vi "DSF.Engine.Transceiver.Initialize.vi"(8 "error in (no error)":errorcluster, 9 "transceiver settings":T1, 10 "Transfer Groups Configurations":refnum<class "DSF.Shared.Configuration.Transfer Group.lvclass">[](array[class]), 11 "Transceiver in":refnum<class "DSF.Transceiver.PXImc.lvclass">) -> (0 "error out":errorcluster, 3 "Transceiver out":refnum<class "DSF.Transceiver.PXImc.lvclass">)   [LabVIEW 2018, in "DSF.Transceiver.PXImc.lvlib" / "DSF.Transceiver.PXImc.lvclass"]
uses:
  DSF.Transceiver.PXImc.lvclass
  dsf core/Built/Engine/DSF.Engine.lvlibp/Shared/Classes/Transfer Group/DSF.Shared.Configuration.Transfer Group.lvclass
  dsf core/Built/Engine/DSF.Engine.lvlibp/DSF Configuration API/1.0.0/Public/Controls/DSF Settings Info.ctl
  DSF.Transceiver.PXImc.lvclass/DSF.Transceiver.PXImc.ctl
  <vilib>/pximc/Initialize Writer Session (U8).vi
  <vilib>/pximc/Connect (U8).vi
  <vilib>/pximc/Initialize Reader Session (U8).vi
  <vilib>/pximc/nipximc.lvlib
  dsf core/Built/Engine/DSF.Engine.lvlibp/DSF Configuration API/1.0.0/DSF Configuration API.lvlib
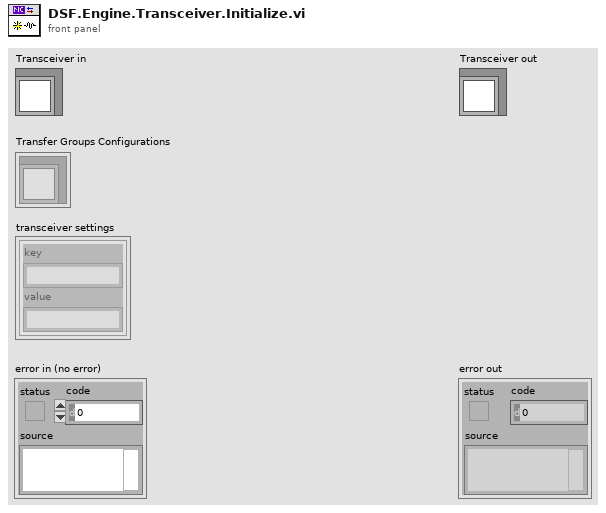
[diagram p1: front panel]
types:
  T1 = typedef "DSF.Engine.lvlibp/DSF Configuration API.lvlib/DSF Settings Info.ctl" = cluster{"key":string, "value":string}[]
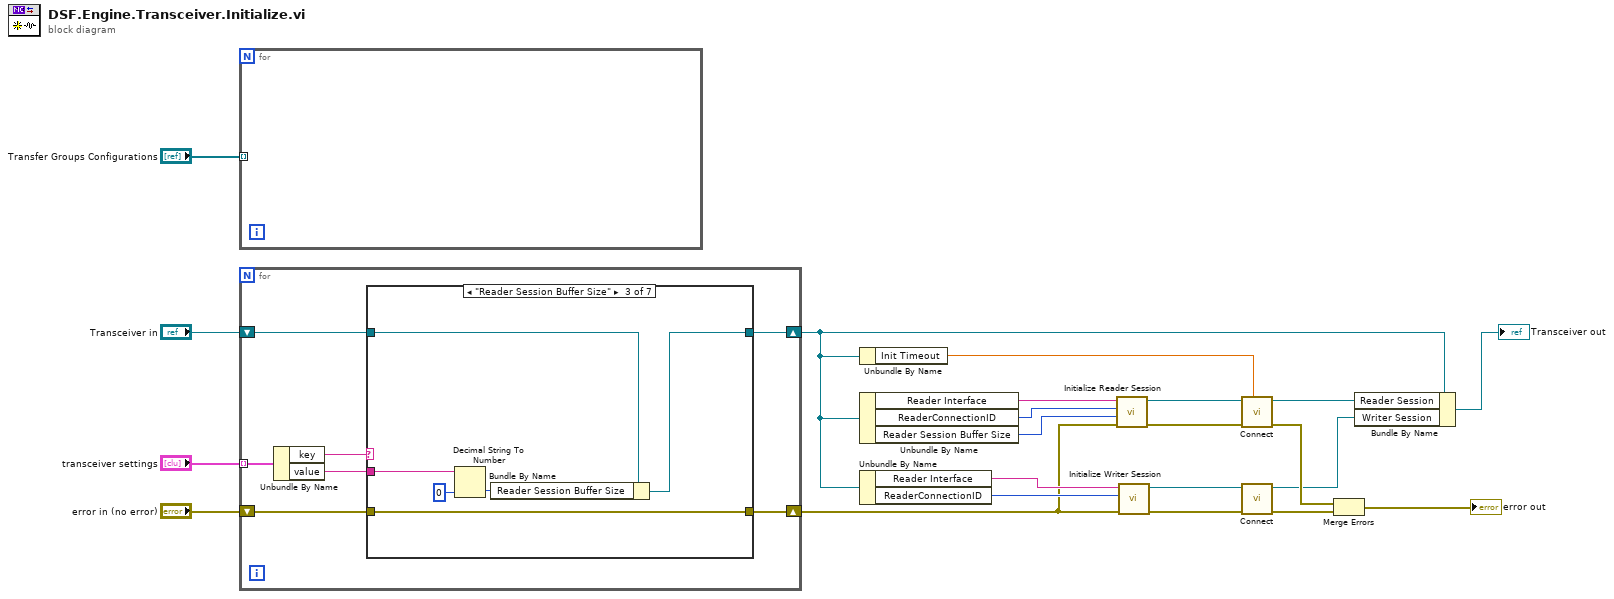
[diagram p0: block diagram]
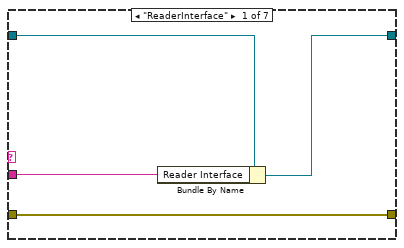
[diagram p2: hidden frame]
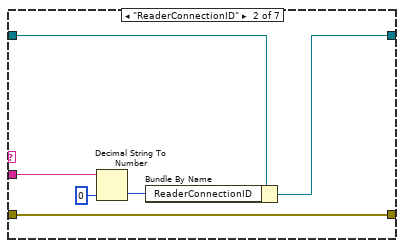
[diagram p3: hidden frame]
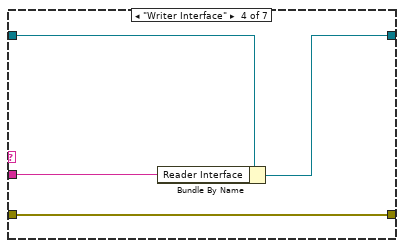
[diagram p4: hidden frame]
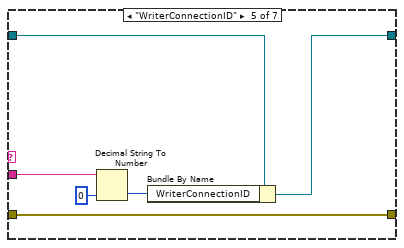
[diagram p5: hidden frame]
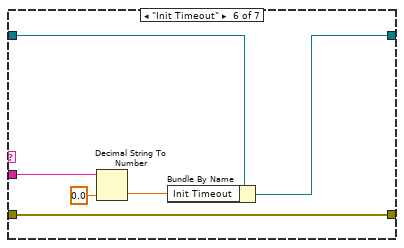
[diagram p6: hidden frame]
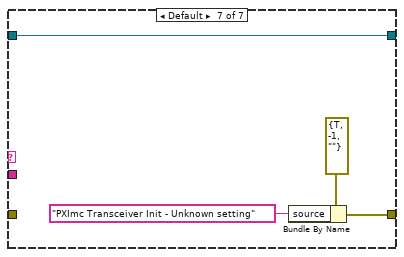
[diagram p7: hidden frame]
diagram:
  n1 = for {
    tunnel: "Transfer Groups Configurations" -> [_] mode=indexing
  }
  n2 = for {
    tunnel: "transceiver settings" -> [w29] mode=indexing
    shift-right: [w25] -> w5
    shift-left: "Transceiver in" -> [w26]
    shift-right: [w23] -> w12
    shift-left: "error in (no error)" -> [w24]
    n3 = Unbundle By Name(w29) -> ("key"=w28:string, "value"=w27:string)
    n4 = case shown="\"Reader Session Buffer Size\"" w28 {
      tunnel: w27 -> [w30 w38 w44 w46 w54 w60 _]
      tunnel: w26 -> [w33 w37 w43 w49 w53 w59 w65]
      tunnel: [w32 w35 w41 w48 w51 w57 w65] -> w25
      tunnel: w24 -> [w31 w34 w40 w47 w50 w56 _]
      tunnel: [w31 w34 w40 w47 w50 w56 w62] -> w23
      frame "ReaderInterface" {
        n5 = Bundle By Name(cluster=w33, "Reader Interface"=w30) -> (w32:refnum<class "DSF.Transceiver.PXImc.lvclass">)
      }
      frame "ReaderConnectionID" {
        n6 = Decimal String To Number(string=w38, default (0L)=u16 0 ("default (0 I32)")) -> (number=w36:u16)  [unwired: 1 in, 1 out]
        n7 = Bundle By Name(cluster=w37, "ReaderConnectionID"=w36) -> (w35:refnum<class "DSF.Transceiver.PXImc.lvclass">)
      }
      frame "Reader Session Buffer Size" {
        n8 = Decimal String To Number(string=w44, default (0L)=u64 0 ("default (0 I32)")) -> (number=w42:u64)  [unwired: 1 in, 1 out]
        n9 = Bundle By Name(cluster=w43, "Reader Session Buffer Size"=w42) -> (w41:refnum<class "DSF.Transceiver.PXImc.lvclass">)
      }
      frame "Writer Interface" {
        n10 = Bundle By Name(cluster=w49, "Reader Interface"=w46) -> (w48:refnum<class "DSF.Transceiver.PXImc.lvclass">)
      }
      frame "WriterConnectionID" {
        n11 = Decimal String To Number(string=w54, default (0L)=u16 0 ("default (0 I32)")) -> (number=w52:u16)  [unwired: 1 in, 1 out]
        n12 = Bundle By Name(cluster=w53, "WriterConnectionID"=w52) -> (w51:refnum<class "DSF.Transceiver.PXImc.lvclass">)
      }
      frame "Init Timeout" {
        n13 = Decimal String To Number(string=w60, default (0L)=0.0 ("default (0 I32)")) -> (number=w58:dbl)  [unwired: 1 in, 1 out]
        n14 = Bundle By Name(cluster=w59, "Init Timeout"=w58) -> (w57:refnum<class "DSF.Transceiver.PXImc.lvclass">)
      }
      frame Default {
        n15 = Bundle By Name(cluster=errorcluster {"status"=TRUE, "code"=-1, "source"=""} ("error constant"), "source"="PXImc Transceiver Init - Unknown setting") -> (w62:errorcluster)
      }
    }
  }
  n16 = Unbundle By Name(w5) -> ("Init Timeout"=w11:dbl)
  n17 = Unbundle By Name(w5) -> ("Reader Interface"=w9:tag, "ReaderConnectionID"=w18:u16, "Reader Session Buffer Size"=w10:u64)
  n18 = Unbundle By Name(w5) -> ("Reader Interface"=w16:tag, "ReaderConnectionID"=w15:u16)
  n19 = call-poly <vilib>:"Initialize Reader Session.vi"("error in (no error)"=w12, "buffer size"=w10, "writer's connection id (1)"=w18, "interface"=w9) -> ("error out"=w17:errorcluster, "session out"=w19:refnum<k21>)  [unwired: 6 in]
  n20 = call-poly <vilib>:"Initialize Writer Session.vi"("error in (no error)"=w12, "connection id (1)"=w15, "interface"=w16) -> ("error out"=w13:errorcluster, "session out"=w14:refnum<k21>)  [unwired: 7 in]
  n21 = call-poly <vilib>:"Connect.vi"("timeout in seconds (-1)"=w11, "error in (no error)"=w17, "session in"=w19) -> ("error out"=w7:errorcluster, "session out"=w4:refnum<k21>)  [unwired: 7 in]
  n22 = call-poly <vilib>:"Connect.vi"("error in (no error)"=w13, "session in"=w14) -> ("error out"=w8:errorcluster, "session out"=w3:refnum<k21>)  [unwired: 8 in]
  n23 = Merge Errors(w7, w8) -> (→"error out":errorcluster)
  n24 = Bundle By Name(cluster=w5, "Reader Session"=w4, "Writer Session"=w3) -> (→"Transceiver out":refnum<class "DSF.Transceiver.PXImc.lvclass">)
